vi "Dashboard Main.vi"() -> ()   [LabVIEW 2017]
uses:
  <vilib>/Utility/miscctls.llb/LVRowAndColumnTypeDef.ctl
  <vilib>/event_ctls.llb/eventvkey.ctl
  <vilib>/Rock Robotics/Network Tables/NT Read Numeric Array.vi
  <vilib>/Rock Robotics/Network Tables/NT Read Boolean Array.vi
  <vilib>/Rock Robotics/WPI/Dashboard/WPI_DashboardLogging Global.vi
panel:
  in  "Camera Settings Right":T1={"Frame Rate"=30, "Compression"=30, "Size"=1, "DB Camera Config"=FALSE} {"Frame Rate" scale=1.0..30.0; "Compression" scale=100.0..-1.0; "Size" items=["640x480", "320x240", "160x120"]}
  in  "Camera Name Right":string(combo)="No Camera Selection"
  out "Camera Info":cluster{"Mbps LED":bool, "Mbps":dbl, "fps":dbl} {"fps" format="%#.1g"; "Mbps" format="%#.1g"}
  in  "Camera Settings":T1={"Frame Rate"=30, "Compression"=30, "Size"=1, "DB Camera Config"=FALSE} {"Frame Rate" scale=1.0..30.0; "Compression" scale=100.0..-1.0; "Size" items=["640x480", "320x240", "160x120"]}
  in  "TCP":refnum<k5>
  in  "Rec Mode":enum32{"Stop", "Record", "Playback"}(radio)
  out "Robot IP":string
  out "Image Message":string="Timeout in Camera Communications"
  in  "Dashboard Tab":T2(tab)
  out "NT Connection":bool
  out "MotorChart R":cluster{"Numeric":dbl, "Numeric":dbl}(graph)
  out "MotorChart L":cluster{"Numeric":dbl, "Numeric":dbl}(graph)
  out "MotorSliders R":cluster{"MotorSlide1":dbl, "MotorSlide2":dbl} {"MotorSlide2" scale=-1.0..1.0 scale format="%#_2e"; "MotorSlide1" scale=-1.0..1.0 scale format="%#_2e"}
  out "MotorSliders L":cluster{"MotorSlide1":dbl, "MotorSlide2":dbl} {"MotorSlide2" scale=-1.0..1.0 scale format="%#_2e"; "MotorSlide1" scale=-1.0..1.0 scale format="%#_2e"}
  out "JS1 Z":dbl(slide) scale=-1.0..1.0 scale format="%#_2e"
  out "JS1 Graph":cluster{"X":dbl, "Y":dbl}[](graph)
  out "JS1 Buttons":T3
  out "JS2 Z":dbl(slide) scale=-1.0..1.0 scale format="%#_2e"
  out "JS2 Graph":cluster{"X":dbl, "Y":dbl}[](graph)
  out "JS2 Buttons":T3
  out "Mode":T4(ring)=enum."Auto Disabled"
  out "Gear State":string="Waiting...."
  out "Ramps":bool[](array[boolean])
  out "Camera Image Right":T5(plugin-control)
  in  "DB/String 9":string
  in  "DB/String 8":string
  in  "DB/String 7":string
  in  "DB/String 6":string
  in  "DB/String 5":string
  in  "DB/String 4":string
  in  "DB/String 3":string
  in  "DB/String 2":string
  in  "DB/String 1":string
  in  "DB/String 0":string
  in  "DB/Slider 0":dbl(slide) scale=0.0..5.0
  in  "DB/Slider 1":dbl(slide) scale=0.0..5.0
  in  "DB/Slider 2":dbl(slide) scale=0.0..5.0
  in  "DB/Slider 3":dbl(slide) scale=0.0..5.0
  out "DB/LED 3":bool
  out "DB/LED 2":bool
  out "DB/LED 1":bool
  out "DB/LED 0":bool
  in  "DB/Button 3":bool
  in  "DB/Button 2":bool
  in  "DB/Button 1":bool
  in  "DB/Button 0":bool caption="New Name"
  in  "Test Slider":dbl(slide) scale=0.0..100.0 scale format="%#_3g"
  in  "On/Off":bool caption="Solenoid"
  in  "Test Name":u16(ring) items=["Select the test to run..."]
  in  "Test Tree":string(tree)
  in  "Motor":cluster{"Value":dbl, "Enable":bool} {"Value" scale=-1.0..1.0 scale format="%#_3g"}
  out "Progress":T6 {"Test Progress" scale=0.0..100.0}
  in  "Rev/Fwd":cluster{"Forward":bool, "Reverse":bool}
  in  "Test Ring":u16(ring) items=["Monochrome", "Color"]
  out "Cmd Status":string
  in  "Execute Command":bool
  in  "Command Params":string[][](table)
  in  "Command Selection":i32(listbox)
  in  "CheckList":i32(listbox)
  out "Tree":string(tree)
  out "new picture":picture
  in  "Starting Pos":i16(slide)=128 scale=340.0..50.0
  in  "Right String":string
  in  "Left String":string
  in  "Load Left Auto":bool
  in  "Save Left Auto":bool
  in  "Save Right Auto":bool
  in  "Load Right Auto":bool
  in  "Select Auto":string(combo)="Select Autonomous ..."
  out "Camera Image":T5(plugin-control)
  out "Background":bool
  in  "Camera Name":string(combo)="No Camera Selection"
  # "HW"
  # "HW"
  # "Joysticks"
  # "Drive Motors"
  # "Front"
  # "Right"
  # "Left"
  # "Back"
  # "This tab is a great place for autonomous settings and robot-specific values.\nPlace controls and indicators inside this tab and match name to\nDashboard Variables on robot. You can also delete this comment."
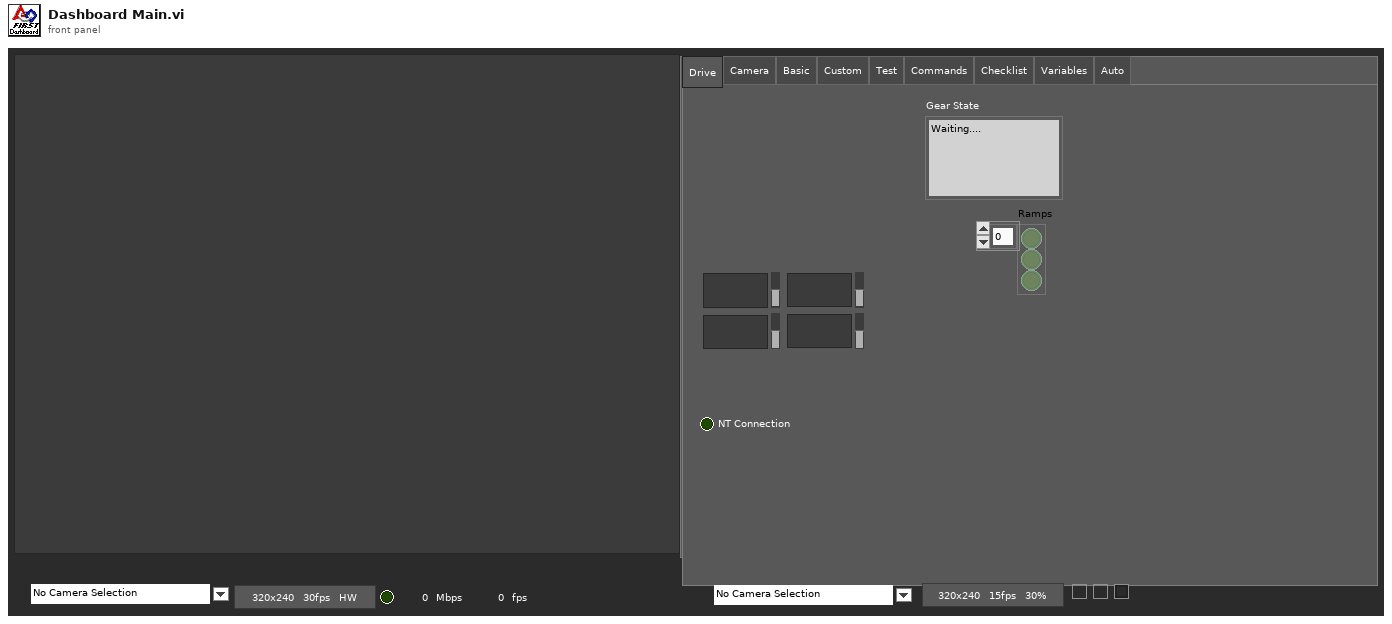
[diagram p1: front panel]
types:
  T1 = cluster{"Frame Rate":i32, "Compression":i32, "Size":u16, "DB Camera Config":bool}
  T2 = enum32{"Drive", "Camera", "Basic", "Custom", "Test", "Commands", "Checklist", "Variables", "Auto"}
  T3 = cluster{bool, bool, bool, bool, bool, bool, bool, bool, bool, bool, bool, bool}
  T4 = enum8{"Tele-Op Disabled", "Tele-Op Enabled", "Auto Disabled", "Auto Enabled", "Test Disabled", "Test Enabled", "Disconnected", "No Code", "E-Stop"}
  T5 = typedef "IMAQ Image.ctl" = refnum<image>
  T6 = cluster{"Test Progress":u8, "Test Progress Text":string}
  T7 = cluster{"Save Path":path, "Interval (s)":dbl, "Keep":i32}
  T8 = enum32{"Drive", "Camera", "Basic", "Custom", "Test", "Commands", "Checklist", "Variables"}
  T9 = typedef "Image Type" = u32
  T10 = cluster{"IDs":cluster{"RPC field ID":u16, "Unique ID":u16}, "String":string}
  T11 = cluster{"Error Strings":string, "Disable Counts":cluster{u16, u16}, "Rail Faults":cluster{u16, u16, u16}, "Robot IP":string, "DB Mode":u8, "Event Info":cluster{"Name":string, "Type":u8, "Number":u16, "Replay":u8}}
  T12 = cluster{"Storage":cluster{"Disk Free":u64, "RAM Block":u32, "RAM free":u32}, "CPU Utilization":cluster{"CPU % ISR":sgl, "CPU % Time Crit":sgl, "CPU % Timed Str":sgl, "CPU % High":sgl, "CPU % Above":sgl, "CPU % Normal":sgl, "CPU % Low":sgl}, "CAN":cluster{"% Bus Utilization":sgl, "Bus Off Cnt":u32, "TX_FIFO Full Cnt":u32, "Receive Error Cnt":u8, "Transmit Error Cnt":u8}, "HID":cluster{"HID Outputs":u32, "Rumble Low":u16, "Rumble High":u16}[]}
  T13 = cluster{"Status bits":cluster{"Test Mode":bool, "Autonomous":bool, "Enabled":bool, "Code Start":bool, "Brownout":bool, "Reserved 2":bool, "Reserved 3":bool, "E-Stop":bool}, "Code Trace":cluster{"Disabled":bool, "TeleOp":bool, "Auto":bool, "Test":bool}, "Controller Type":enum16{"unknown", "cRIO", "roboRio"}, "Code?":enum16{"unknown", "noCode", "code"}, "Battery V":dbl}
  T14 = cluster{"Control Bits":cluster{"TestMode":bool, "Autonomous":bool, "Enabled":bool, "FMS Present":bool, bool, bool, bool, "E-Stop":bool}, "Team Station ":u8, "Countdown":sgl, "Joystick Values":cluster{"Axes":dbl[], "Buttons":bool[], "POVs":i16[]}[]}
  T15 = cluster{"Axes":dbl[], "Buttons":bool[], "POVs":i16[]}[]
  T16 = cluster{"Axes":dbl[], "Buttons":bool[], "POVs":i16[]}
  T17 = cluster{"Buttons[0]":bool, "Buttons[1]":bool, "Buttons[2]":bool, "Buttons[3]":bool, "Buttons[4]":bool, "Buttons[5]":bool, "Buttons[6]":bool, "Buttons[7]":bool, "Buttons[8]":bool, "Buttons[9]":bool, "Buttons[10]":bool, "Buttons[11]":bool}
  T18 = typedef "LVBoundsTypeDef.ctl" = cluster{"Width":u32, "Height":u32}
  T19 = cluster{"Camera Image":refnum<vi>, "Dashboard Tab":refnum<vi>, "Background":refnum<vi>, "Rec Mode":refnum<vi>, "Test Slider":refnum<vi>, "On/Off ":refnum<vi>, "Test Ring":refnum<vi>, "Rev/Fwd":refnum<vi>, "Test Name":refnum<vi>, "Motor":refnum<vi>, "Progress":refnum<vi>, "CheckList":refnum<vi>, "Tree":refnum<vi>, "Test Tree":refnum<vi>, "Command Params":refnum<vi>, "Command Selection":refnum<vi>, "Execute Command":refnum<vi>, "Cmd Status":refnum<vi>, "Camera Settings":refnum<vi>, "Camera Name":refnum<vi>, "Camera Info":refnum<vi>, "Camera Settings Right":refnum<vi>, "Camera Name Right":refnum<vi>, "Camera Image Right":refnum<vi>}
  T20 = cluster{"Camera Name":string, string, "Saved DB Images Info":cluster{"Save Path":path, "Interval (s)":dbl, "Keep":i32}}
  T21 = cluster{"Camera Name Right":string, string, "Saved DB Images Info":cluster{"Save Path":path, "Interval (s)":dbl, "Keep":i32}}
  T22 = cluster{"Operation":enum16{"Update", "Clear"}, "Color Box":u32}[]
  T23 = typedef "eventvkey.ctl" = enum16{"ASCII", "Enter", "Return", "Shift", "Ctrl", "Alt", "Cmd", "Opt", "Caps", "NumLock", "Clear", "Break", "Up", "Down", "Left", "Right", "Insert", "Delete", "Home", "End", "PageUp", "PageDown", "Escape", "Help", "Pause", "ScrollLock", "F1", "F2", "F3", "F4", "F5", "F6", "F7", "F8", "F9", "F10", "F11", "F12", "F13", "F14", "F15", "F16", "F17", "F18", "F19", "F20", "F21", "F22", "F23", "F24", "Play", "VolumeUp", "VolumeDown", "Mute", "Two Byte Char"}
  T24 = cluster{"Image Size":bool, "Image Type":bool, "Pixel Value":bool, "ROI Information":bool, "Zoom Factor":bool}
  T25 = cluster{"Operation":enum16{"Update", "Clear"}, "Color Box":u32}
  T26 = typedef "LVRowAndColumnTypeDef.ctl" = cluster{"Row":i32, "Column":i32}
  T27 = cluster{"Shift":bool, "Ctrl":bool, "Alt":bool, "Cmd":bool, "Opt":bool}
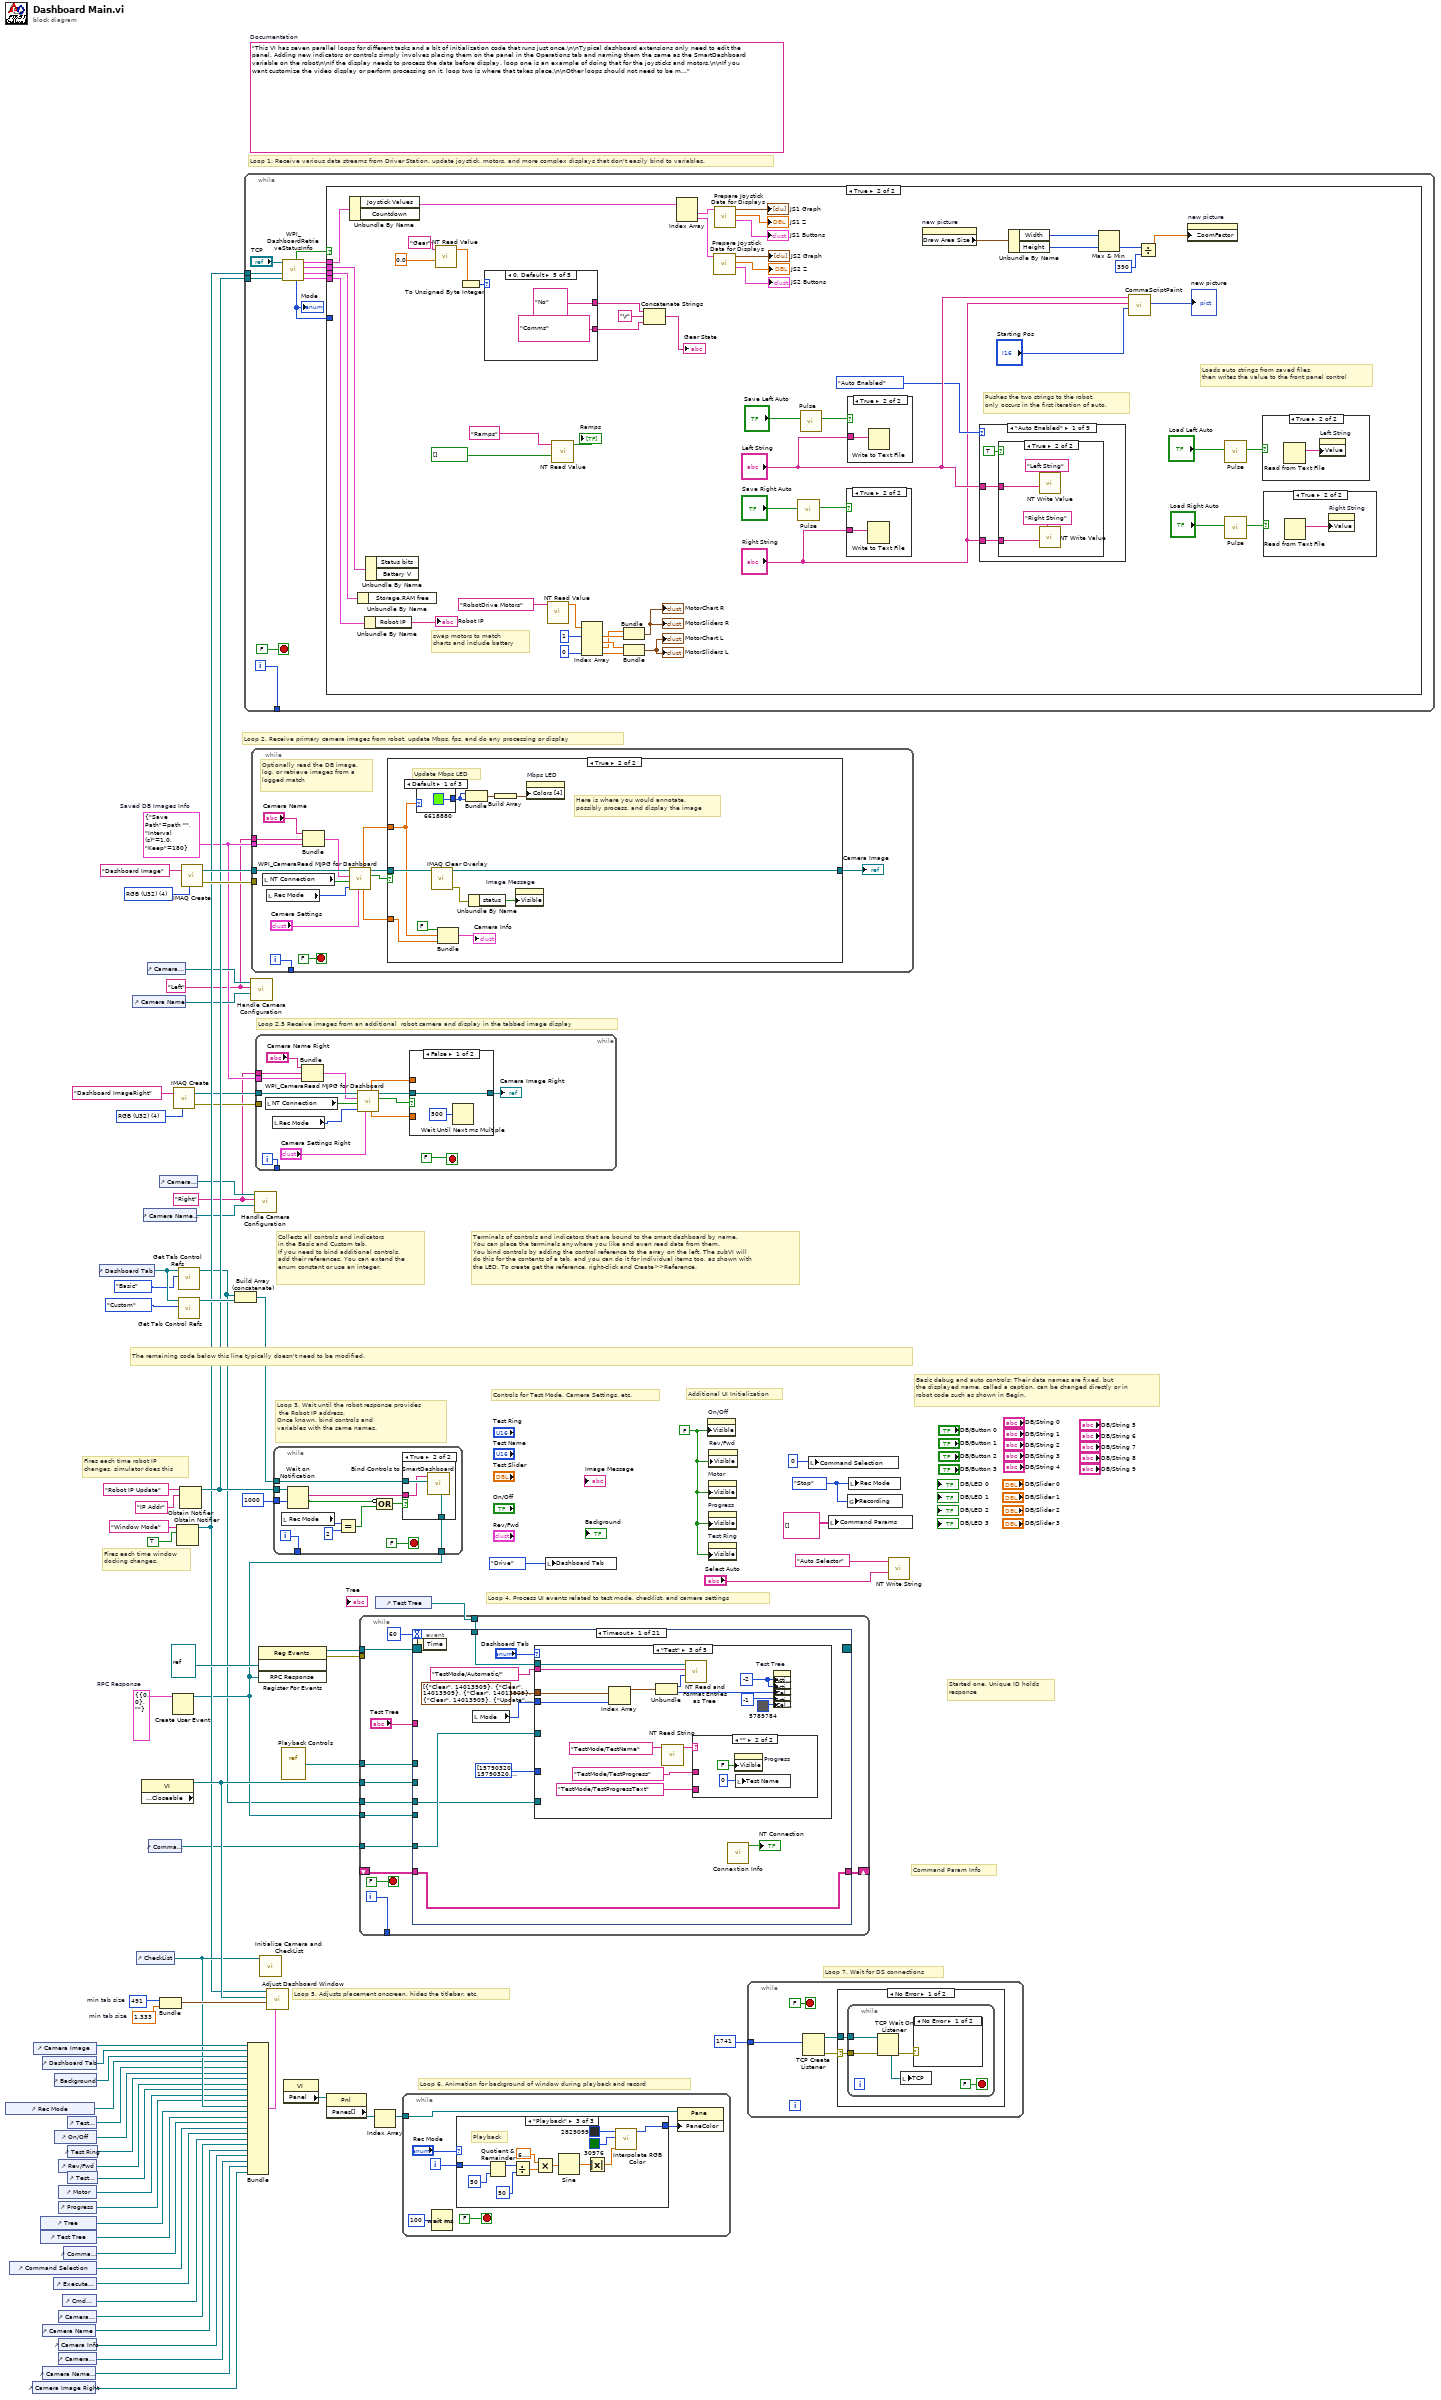
[diagram p0: block diagram]
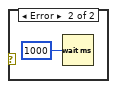
[diagram p3: hidden frame]
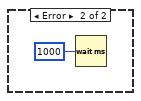
[diagram p4: hidden frame]
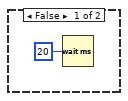
[diagram p5: hidden frame]
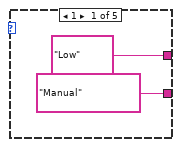
[diagram p19: hidden frame]
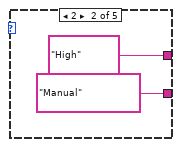
[diagram p20: hidden frame]
diagram:
  w3 = T7 {"Save Path"=path "", "Interval (s)"=1.0, "Keep"=180}  # Saved DB Images Info
  w2 = "Right"
  w1 = "Left"
  w13 = T9 4 items=["Grayscale (U8)", "Grayscale (I16)", "Grayscale (SGL)", "Complex (CSG)", "RGB (U32)", "HSL (U32)", "RGB (U64)"] ("Image Type")
  w29 = T10 {"IDs"={"RPC field ID"=0, "Unique ID"=0}, "String"=""}  # RPC Response
  w52 = 491  # min tab size
  w51 = 1.333  # min tab size
  w59 = enum32{"Stop", "Record", "Playback"}."Stop" ("Rec Mode")
  w36 = FALSE ("Visible")
  (unwired) "This VI has seven parallel loops for different tasks and a bit of initialization code that runs just once.\n\nTypical dashboard extensions only need to edit the panel. Adding new indicators or controls simply involves placing them on the panel in the Operations tab and naming them the same as the SmartDashboard variable on the robot\n\nIf the display needs to process the data before display, loop one is an example of doing that for the joysticks and motors.\n\nIf you want customize the video display or perform processing on it, loop two is where that takes place.\n\nOther loops should not need to be modified. They are pretty standard, and document the task they perform."  # Documentation
  w76 = T9 4 items=["Grayscale (U8)", "Grayscale (I16)", "Grayscale (SGL)", "Complex (CSG)", "RGB (U32)", "HSL (U32)", "RGB (U64)"] ("Image Type")
  # "Loop 2.5 Receive images from an additional  robot camera and display in the tabbed image display"
  # "Command Param Info"
  # "Started one, Unique ID holds\nresponse"
  # "Loop 7. Wait for DS connections"
  # "Basic debug and auto controls: Their data names are fixed, but\nthe displayed name, called a caption, can be changed directly or in\nrobot code such as shown in Begin."
  # "Controls for Test Mode, Camera Settings, etc."
  # "Additional UI Initialization"
  # "Loop 6. Animation for background of window during playback and record"
  # "Fires each time robot IP\nchanges, simulator does this"
  # "Fires each time window\ndocking changes."
  # "Collects all controls and indicators\nin the Basic and Custom tab.\nIf you need to bind additional controls,\nadd their references. You can extend the\nenum constant or use an integer."
  # "The remaining code below this line typically doesn't need to be modified."
  # "Loop 4. Process UI events related to test mode, checklist, and camera settings"
  # "Terminals of controls and indicators that are bound to the smart dashboard by name.\nYou can place the terminals anywhere you like and even read data from them.\nYou bind controls by adding the control reference to the array on the left. The subVI will\ndo this for the contents of a tab, and you can do it for individual items too, as shown with\nthe LED. To create get the reference, right-click and Create>>Reference."
  # "Loop 3. Wait until the robot response provides\n the Robot IP address.\nOnce known, bind controls and\nvariables with the same names."
  # "Loop 5. Adjusts placement onscreen, hides the titlebar, etc."
  # "Loop 1. Receive various data streams from Driver Station, update joystick, motors, and more complex displays that don't easily bind to variables."
  # "Loop 2. Receive primary camera images from robot, update Mbps, fps, and do any processing or display"
  n1 = control-ref of="Rec Mode"() -> (w42:refnum<vi>)
  n2 = control-ref of="Command Selection"() -> (w28:refnum<vi>)
  n3 = control-ref of="Camera Image Right"() -> (w6:refnum<vi>)
  n4 = control-ref of="Camera Image"() -> (w54:refnum<vi>)
  n5 = control-ref of="Tree"() -> (w46:refnum<vi>)
  n6 = control-ref of="Test Tree"() -> (w45:refnum<vi>)
  n7 = control-ref of="Dashboard Tab"() -> (w53:refnum<vi>)
  n8 = control-ref of="Camera Name"() -> (w19:refnum<vi>)
  n9 = control-ref of="Camera Name Right"() -> (w7:refnum<vi>)
  n10 = control-ref of="Execute Command"() -> (w30:refnum<vi>)
  n11 = control-ref of="Background"() -> (w49:refnum<vi>)
  n12 = control-ref of="On/Off"() -> (w40:refnum<vi>)
  n13 = control-ref of="Progress"() -> (w37:refnum<vi>)
  n14 = control-ref of="Camera Settings"() -> (w20:refnum<vi>)
  n15 = control-ref of="Camera Info"() -> (w18:refnum<vi>)
  n16 = control-ref of="Camera Settings Right"() -> (w8:refnum<vi>)
  n17 = control-ref of="Rev/Fwd"() -> (w38:refnum<vi>)
  n18 = control-ref of="Motor"() -> (w43:refnum<vi>)
  n19 = control-ref of="Cmd Status"() -> (w24:refnum<vi>)
  n20 = control-ref of="Command Params"() -> (w31:refnum<vi>)
  n21 = control-ref of="Test Slider"() -> (w41:refnum<vi>)
  n22 = control-ref of="Test Ring"() -> (w39:refnum<vi>)
  n23 = control-ref of="Test Name"() -> (w44:refnum<vi>)
  n24 = control-ref of="Dashboard Tab"() -> (w57:refnum<vi>)
  n25 = control-ref of="Camera Name"() -> (w21:refnum<vi>)
  n26 = control-ref of="CheckList"() -> (w47:refnum<vi>)
  n27 = property class="VI" props=["Front Panel.Closeable"]() -> (reference out=w58:refnum<vi>)  [unwired: 2 in, 2 out]
  n28 = control-ref of="Camera Name Right"() -> (w9:refnum<vi>)
  n29 = control-ref of="Camera Settings"() -> (w22:refnum<vi>)
  n30 = control-ref of="Command Params"() -> (w23:refnum<vi>)
  n31 = control-ref of="Camera Settings Right"() -> (w10:refnum<vi>)
  n32 = Bundle("min tab size"=w52, "min tab size"=w51) -> (w50:cluster{"min tab size":i32, "min tab size":dbl})  [unwired: 1 in]
  n33 = Create User Event(user event datatype=w29) -> (user event=w25:refnum<user-event>)  [unwired: 1 in, 1 out]
  n34 = call "IMAQ Create"("Image Name"="Dashboard ImageRight", "Image Type"=w13) -> ("New Image"=w12:T5, "error out"=w11:errorcluster)  [unwired: 2 in, 1 out]
  n35 = Obtain Notifier(name (unnamed)="Window Mode", notification data type=TRUE) -> (notifier out=w34:refnum<notifier>)  [unwired: 2 in, 2 out]
  n36 = call <vilib>:"Get Tab Control Refs.vi"("Page Index"=T8."Basic" ("Dashboard Tab"), "TabControl in"=w57) -> ("ControlsOnPage"=w17:refnum<vi>[])  [unwired: 9 in]
  n37 = call <vilib>:"Get Tab Control Refs.vi"("Page Index"=T8."Custom" ("Dashboard Tab"), "TabControl in"=w57) -> ("ControlsOnPage"=w56:refnum<vi>[])  [unwired: 9 in]
  n38 = Obtain Notifier(name (unnamed)="Robot IP Update", notification data type="IP Addr" ("name (unnamed)")) -> (notifier out=w35:refnum<notifier>)  [unwired: 2 in, 2 out]
  n39 = call "IMAQ Create"("Image Name"="Dashboard Image", "Image Type"=w76) -> ("New Image"=w74:T5, "error out"=w73:errorcluster)  [unwired: 2 in, 1 out]
  n40 = Build Array (concatenate)(w17, w56) -> (w55:refnum<vi>[])
  n41 = while {
    tunnel: [w86] -> _
    tunnel: w35 -> [w80]
    tunnel: w34 -> [w77]
    i -> [w86]
    stop <- FALSE stop-if-true
    n42 = call <vilib>:"WPI_DashboardRetrieveStatusInfo.vi"("Binding Refnum"=w80, "Window Mode Notifier"=w77, "TCP Cnx"="TCP") -> ("Power and Errors"=w81:T11, "Robot Metrics"=w84:T12, "Status Info"=w85:T13, "Control Info"=w82:T14, "Robot Mode"=w79:T4, "Process?"=w83:bool)  [unwired: 3 in]
    "Mode" <- w79
    n43 = case shown="True" w83 {
      tunnel: w85 -> [_ w142]
      tunnel: w84 -> [_ w141]
      tunnel: w82 -> [_ w140]
      tunnel: w81 -> [_ w139]
      tunnel: w79 -> [_ _]
      frame False {
        n44 = Wait (ms)(milliseconds to wait=u32 20) -> ()  [unwired: 1 out]
      }
      frame True {
        # "Pushes the two strings to the robot,\nonly occurs in the first iteration of auto."
        # "Loads auto strings from saved files,\nthen writes the value to the front panel control"
        # "swap motors to match\ncharts and include battery"
        n45 = Unbundle By Name(w140) -> ("Joystick Values"=w130:T15)  [unwired: 1 out]
        n46 = Unbundle By Name(w141) -> ()  [unwired: 1 out]
        n47 = Unbundle By Name(w139) -> ("Robot IP"=→"Robot IP":string)
        n48 = Unbundle By Name(w142) -> ()  [unwired: 2 out]
        n49 = call-poly <vilib>:"NT Read Value.vi"("Default Value"=0.0, "Name"="Gear") -> ("Numeric"=w117:dbl)  [unwired: 8 in, 1 out]
        n50 = To Unsigned Byte Integer(number=w117) -> (unsigned 8bit integer=w118:u8)
        n51 = case shown="0, Default" w118 {
          tunnel: ["Low" "High" "Low" "High" "No"] -> w114
          tunnel: ["Manual" "Manual" "Automatic" "Automatic" "Comms"] -> w112
          frame 1 {
          }
          frame 2 {
          }
          frame 3 {
          }
          frame 4 {
          }
          frame 0, Default {
          }
        }
        n52 = call-poly <vilib>:"NT Read Value.vi"("Name"="RobotDrive Motors") -> ("Numeric Array"=w120:dbl[])  [unwired: 9 in, 1 out]
        n53 = call-poly <vilib>:"NT Read Value.vi"("Default Value"=bool[] [], "Name"="Ramps") -> ("Boolean Array"=→"Ramps":bool[])  [unwired: 8 in, 1 out]
        n54 = Index Array(array=w120, index #1=1, index #4=0) -> (element #1=w134:dbl, element #2=w135:dbl, element #3=w133:dbl, element #4=w138:dbl)  [unwired: 2 in]
        n55 = Bundle("Numeric"=w133, "Numeric"=w134) -> (→"MotorChart R" →"MotorSliders R":cluster{"Numeric":dbl, "Numeric":dbl})  [unwired: 1 in]
        n56 = Bundle("Numeric"=w135, "Numeric"=w138) -> (→"MotorChart L" →"MotorSliders L":cluster{"Numeric":dbl, "Numeric":dbl})  [unwired: 1 in]
        n57 = Concatenate Strings(w114, "\r", w112) -> (→"Gear State":string)
        n58 = Index Array(array=w130) -> (element #1=w129:T16, element #2=w125:T16)  [unwired: 2 in]
        n59 = call "Prepare Joystick Data for Displays.vi"("Joystick Values"=w125) -> ("Buttons"=→"JS2 Buttons":T17, "Z Axis"=→"JS2 Z":dbl, "Cartesian Data"=→"JS2 Graph":cluster{"X axis":dbl, "X axis":dbl}[])  [unwired: 8 in]
        n60 = call "Prepare Joystick Data for Displays.vi"("Joystick Values"=w129) -> ("Buttons"=→"JS1 Buttons":T17, "Z Axis"=→"JS1 Z":dbl, "Cartesian Data"=→"JS1 Graph":cluster{"X axis":dbl, "X axis":dbl}[])  [unwired: 8 in]
        n61 = call "Pulse.vi"("Input"="Save Right Auto") -> ("Output"=w105:bool)  [unwired: 10 in]
        n62 = call "Pulse.vi"("Input"="Save Left Auto") -> ("Output"=w101:bool)  [unwired: 10 in]
        n63 = case shown="True" w105 {
          tunnel: "Right String" -> [_ w150]
          frame False {
          }
          frame True {
            n64 = Write to Text File(text=w150) -> ()  [unwired: 3 in, 3 out]
          }
        }
        n65 = case shown="True" w101 {
          tunnel: "Left String" -> [_ w153]
          frame False {
          }
          frame True {
            n66 = Write to Text File(text=w153) -> ()  [unwired: 3 in, 3 out]
          }
        }
        n67 = property on="new picture" class="Pict"() -> ("Draw Area Size"=w93:T18)  [unwired: 2 in, 2 out]
        n68 = case shown="\"Auto Enabled\"" T4."Auto Enabled" ("Robot Mode") {
          tunnel: "Left String" -> [w145 _ _ _ _ _ _ _ _]
          tunnel: "Right String" -> [w144 _ _ _ _ _ _ _ _]
          frame "Auto Enabled" {
            n69 = case shown="True" TRUE {
              tunnel: w145 -> [_ w149]
              tunnel: w144 -> [_ w148]
              frame False {
              }
              frame True {
                n70 = call-poly <vilib>:"NT Write Value.vi"("String"=w149, "Name"="Left String") -> ()  [unwired: 9 in, 1 out]
                n71 = call-poly <vilib>:"NT Write Value.vi"("String"=w148, "Name"="Right String") -> ()  [unwired: 9 in, 1 out]
              }
            }
          }
          frame "Test Disabled" {
          }
          frame "Test Enabled" {
          }
          frame "Disconnected" {
          }
          frame "No Code" {
          }
          frame "E-Stop" {
          }
          frame "Auto Disabled" {
          }
          frame "Tele-Op Enabled" {
          }
          frame "Tele-Op Disabled" {
          }
        }
        n72 = Unbundle By Name(w93) -> ("Width"=w97:u32, "Height"=w96:u32)
        n73 = Max & Min(x=w97, y=w96) -> (min(x,y)=w95:u32)  [unwired: 1 out]
        n74 = call "CommaScriptPaint.vi"("Starting Pos"="Starting Pos", "string 2"="Right String", "string"="Left String") -> ("new picture"=→"new picture":picture)  [unwired: 7 in, 1 out]
        n75 = Divide(x=w95, y=u32 390) -> (x/y=w92:dbl)
        n76 = property on="new picture" class="Pict"("ZoomFactor"=w92) -> ()  [unwired: 2 in, 2 out]
        n77 = call "Pulse.vi"("Input"="Load Left Auto") -> ("Output"=w102:bool)  [unwired: 10 in]
        n78 = call "Pulse.vi"("Input"="Load Right Auto") -> ("Output"=w108:bool)  [unwired: 10 in]
        n79 = case shown="True" w102 {
          frame False {
          }
          frame True {
            n80 = Read from Text File() -> (text=w152:string)  [unwired: 4 in, 3 out]
            n81 = property on="Left String" class="Str"("Value"=w152) -> ()  [unwired: 2 in, 2 out]
          }
        }
        n82 = case shown="True" w108 {
          frame False {
          }
          frame True {
            n83 = Read from Text File() -> (text=w151:string)  [unwired: 4 in, 3 out]
            n84 = property on="Right String" class="Str"("Value"=w151) -> ()  [unwired: 2 in, 2 out]
          }
        }
      }
    }
  }
  n85 = Bundle("Camera Image"=w54, "Dashboard Tab"=w53, "Background"=w49, "Rec Mode"=w42, "Test Slider"=w41, "On/Off"=w40, "Test Ring"=w39, "Rev/Fwd"=w38, "Test Name"=w44, "Motor"=w43, "Progress"=w37, "CheckList"=w47, "Tree"=w46, "Test Tree"=w45, "Command Params"=w31, "Command Selection"=w28, "Execute Command"=w30, "Cmd Status"=w24, "Camera Settings"=w20, "Camera Name"=w19, "Camera Info"=w18, "Camera Settings Right"=w8, "Camera Name Right"=w7, "Camera Image Right"=w6) -> (w48:T19)  [unwired: 1 in]
  n86 = call "Handle Camera Configuration.vi"("CameraNameRef"=w21, "Display Name"=w1, "ClusterRef"=w22) -> ()  [unwired: 9 in]
  n87 = while {
    tunnel: w74 -> [w176]
    tunnel: w73 -> [_]
    tunnel: [w177] -> _
    tunnel: w3 -> [w167]
    tunnel: w1 -> [w164]
    i -> [w177]
    stop <- FALSE stop-if-true
    # "Optionally read the DB image,\nlog, or retrieve images from a\nlogged match"
    n88 = local read "NT Connection"() -> (w168:bool)
    n89 = local read "Rec Mode"() -> (w172:enum32{"Stop", "Record", "Playback"})
    n90 = Bundle("Camera Name"="Camera Name", w164, "Saved DB Images Info"=w167) -> (w166:T20)  [unwired: 1 in]
    n91 = call <vilib>:"WPI_CameraRead MJPG for Dashboard.vi"("Camera Settings"="Camera Settings", "Rec Mode"=w172, "NT Connection"=w168, "Capture Info"=w166, "Refnum in"=w176) -> ("Active"=w174:bool, "Refnum out"=w175:T5, "FPS"=w173:dbl, "Bandwidth (Mbps)"=w171:dbl)  [unwired: 3 in]
    n92 = case shown="True" w174 {
      tunnel: w175 -> [w179 w190]
      tunnel: w171 -> [_ w187]
      tunnel: w173 -> [_ w188]
      tunnel: [w179 w184] -> w169
      frame False {
        w181 = u32 1985280 ("Color Box")
        # "Sleep for 500ms"
        n93 = Bundle("Color Box"=w181, "Color Box"=w181) -> (w182:cluster{"Color Box":u32, "Color Box":u32})  [unwired: 1 out]
        n94 = Build Array(w182) -> (w180:cluster{"Color Box":u32, "Color Box":u32}[])
        n95 = property on="Mbps LED" class="Bool (strict)"("Colors [4]"=w180) -> ()  [unwired: 2 in, 2 out]
        n96 = Wait Until Next ms Multiple(millisecond multiple=u32 500) -> ()  [unwired: 1 out]
      }
      frame True {
        # "Here is where you would annotate,\npossibly process, and display the image"
        # "Update Mbps LED"
        n97 = case shown="Default" w187 {
          tunnel: [u32 6618880 ("Color Box") u32 16776722 ("Color Box") u32 16716800 ("Color Box")] -> w191
          frame Default {
          }
          frame 4, 5 {
          }
          frame 6.. {
          }
        }
        n98 = call "IMAQ Clear Overlay"("Image"=w190) -> ("error out"=w193:errorcluster, "Image Out"=w184:T5)  [unwired: 2 in, 7 out]
        n99 = Bundle(FALSE, "Bandwidth (Mbps)"=w187, "FPS"=w188) -> (→"Camera Info":cluster{bool, "Bandwidth (Mbps)":dbl, "FPS":dbl})  [unwired: 1 in]
        n100 = Bundle("Color Box"=w191, "Color Box"=w191) -> (w192:cluster{"Color Box":u32, "Color Box":u32})  [unwired: 1 out]
        n101 = Unbundle By Name(w193) -> ("status"=w194:bool)
        n102 = Build Array(w192) -> (w189:cluster{"Color Box":u32, "Color Box":u32}[])
        n103 = property on="Image Message" class="Str"("Visible"=w194) -> ()  [unwired: 2 in, 2 out]
        n104 = property on="Mbps LED" class="Bool (strict)"("Colors [4]"=w189) -> ()  [unwired: 2 in, 2 out]
      }
    }
    "Camera Image" <- w169
  }
  n105 = call "Handle Camera Configuration.vi"("CameraNameRef"=w9, "Display Name"=w2, "ClusterRef"=w10) -> ()  [unwired: 9 in]
  n106 = while {
    tunnel: w12 -> [w212]
    tunnel: w11 -> [_]
    tunnel: [w207] -> _
    tunnel: w3 -> [w201]
    tunnel: w2 -> [w198]
    i -> [w207]
    stop <- FALSE stop-if-true
    n107 = local read "NT Connection"() -> (w202:bool)
    n108 = local read "Rec Mode"() -> (w211:enum32{"Stop", "Record", "Playback"})
    n109 = Bundle("Camera Name Right"="Camera Name Right", w198, "Saved DB Images Info"=w201) -> (w200:T21)  [unwired: 1 in]
    n110 = call <vilib>:"WPI_CameraRead MJPG for Dashboard.vi"("Camera Settings"="Camera Settings Right", "Rec Mode"=w211, "NT Connection"=w202, "Capture Info"=w200, "Refnum in"=w212) -> ("Active"=w206:bool, "Refnum out"=w209:T5, "FPS"=w204:dbl, "Bandwidth (Mbps)"=w205:dbl)  [unwired: 3 in]
    n111 = case shown="False" w206 {
      tunnel: w209 -> [w213 w215]
      tunnel: w205 -> [_ _]
      tunnel: w204 -> [_ _]
      tunnel: [w213 w215] -> w203
      frame False {
        n112 = Wait Until Next ms Multiple(millisecond multiple=u32 500) -> ()  [unwired: 1 out]
      }
      frame True {
      }
    }
    "Camera Image Right" <- w203
  }
  n113 = register-events(refnum<vi> refnum, w25) -> (reference out=w63:refnum<event-registration>, error out=w62:errorcluster)  [unwired: 2 in]
  n114 = call "Initialize Camera and CheckList.vi"("ListBox in"=w47) -> ()  [unwired: 11 in]
  n115 = call "Adjust Dashboard Window.vi"("Sizing Refnums"=w48, "Size Constraints"=w50, "VI"=w58, "WIn Mode"=w34) -> ()  [unwired: 8 in]
  n116 = while {
    tunnel: w55 -> [w227]
    tunnel: w35 -> [w225]
    tunnel: [w223] -> _
    tunnel: u32 1000 ("milliseconds to wait") -> [w222]
    tunnel: w25 -> [w216]
    i -> [w223]
    stop <- FALSE stop-if-true
    n117 = local read "Rec Mode"() -> (w218:enum32{"Stop", "Record", "Playback"})
    n118 = Wait on Notification(notifier=w225, timeout in ms (-1)=w222) -> (notification=w224:string, timed out?=w220:bool)  [unwired: 2 in, 2 out]
    n119 = Equal?(x=w218, y=u16 2 ("Rec Mode")) -> (x = y?=w219:bool)
    n120 = Compound Arithmetic op=OR(invert w220, w219) -> (w221:bool)
    n121 = case shown="True" w221 {
      tunnel: w227 -> [_ w230]
      tunnel: w224 -> [_ w229]
      tunnel: w216 -> [_ w228]
      frame False {
      }
      frame True {
        n122 = call <vilib>:"Bind Controls to SmartDashboard.vi"("RPC ref"=w228, "Bound Control Refs"=w230, "Server IP Address"=w229) -> ()  [unwired: 9 in]
      }
    }
  }
  n123 = vi-ref "Playback Controls.vi"() -> (w64:refnum<vi>)
  n124 = property class="VI"() -> ("Panel"=w66:refnum<vi>)  [unwired: 2 in, 2 out]
  n125 = property class="Pnl"(reference=w66) -> ("Panes[]"=w67:refnum<vi>[])  [unwired: 1 in, 2 out]
  n126 = Index Array(array=w67) -> (element=w65:refnum<vi>)  [unwired: 1 in]
  n127 = control-ref of="Test Tree"() -> (w68:refnum<vi>)
  n128 = while {
    tunnel: [w240] -> _
    tunnel: w68 -> [w239]
    tunnel: w64 -> [w238]
    tunnel: w63 -> [w237]
    tunnel: w62 -> [_]
    tunnel: w58 -> [w236]
    tunnel: w25 -> [w235]
    tunnel: w23 -> [w234]
    shift-right: [w233] -> _
    shift-left: _ -> [w232]
    tunnel: w17 -> [w231]
    i -> [w240]
    stop <- FALSE stop-if-true
    n129 = event shown="[0] Timeout" {
      selector: w237 -> [_ _ _ _ _ _ _ _ _ _ _ _ _ _ _ _ _ _ _ _ _]
      dyn-events: [_ _ _ _ _ _ _ _ _ _ _ _ _ _ _ _ w500 _ _ _ _] -> _
      timeout: u32 60 ("milliseconds to wait") -> [_ _ _ _ _ _ _ _ _ _ _ _ _ _ _ _ _ _ _ _ _]
      tunnel: w239 -> [w252 _ _ _ _ _ _ _ _ _ _ _ _ _ _ _ _ _ _ _ _]
      tunnel: "Test Tree" -> [_ _ _ _ _ _ _ _ _ _ _ w467 w475 w477 w481 w489 _ _ _ _ _]
      tunnel: w238 -> [_ _ _ _ _ _ _ _ _ _ _ _ _ _ _ _ w502 _ w520 _ _]
      tunnel: w236 -> [_ _ _ _ _ _ _ _ _ _ _ _ _ _ _ _ w498 _ _ _ _]
      tunnel: w235 -> [_ _ _ _ _ _ _ _ _ _ _ _ _ _ _ _ w496 _ _ _ _]
      tunnel: w234 -> [w247 _ _ _ _ _ w418 _ _ _ _ _ _ _ _ _ _ _ _ _ _]
      tunnel: [w246 w295 w397 w402 w411 w415 w416 w425 w435 w442 w454 w466 w473 w476 w480 w488 w495 w515 w517 w521 w534] -> w233
      tunnel: w232 -> [w246 w295 w397 w402 w411 w415 w416 _ _ w442 w454 w466 w473 w476 w480 w488 w495 w515 w517 w521 w534]
      tunnel: w231 -> [w244 _ _ _ _ _ _ _ _ _ _ _ _ _ _ _ _ _ _ _ _]
      event Timeout {
        n130 = event-data() -> ()  [unwired: 1 in, 1 out]
        n131 = local read "Mode"() -> (w249:T4)
        n132 = case shown="\"Test\"" "Dashboard Tab" {
          tunnel: w252 -> [_ _ w268 _ _]
          tunnel: "TestMode/Automatic/" ("Name Pattern") -> [_ _ w267 _ _]
          tunnel: T22 [{"Operation"=enum."Clear", "Color Box"=14013909}, {"Operation"=enum."Clear", "Color Box"=14013909}, {"Operation"=enum."Clear", "Color Box"=14013909}, {"Operation"=enum."Clear", "Color Box"=14013909}, {"Operation"=enum."Update", "Color Box"=14013909}, {"Operation"=enum."Update", "Color Box"=16777215}, {"Operation"=enum."Clear", "Color Box"=14013909}, {"Operation"=enum."Clear", "Color Box"=14013909}, {"Operation"=enum."Clear", "Color Box"=14013909}] -> [_ _ w260 _ w288]
          tunnel: w249 -> [_ _ w259 _ w287]
          tunnel: u32[] [15790320, 15790320, 15790320, 15790320, 16777215, 16777215, 15790320, 15790320, 15790320] -> [_ _ _ _ w293]
          tunnel: w247 -> [_ _ _ _ w281]
          tunnel: w244 -> [_ w254 _ _ _]
          frame "Custom", Default {
          }
          frame "Basic" {
            n133 = call <vilib>:"WPI_DashboardUpdateNames.vi"("Controls on Tab"=w254) -> ()  [unwired: 11 in]
          }
          frame "Test" {
            w266 = -2 ("Active Item:Row Number")
            n134 = Index Array(array=w260, index=w259) -> (element=w261:T25)
            n135 = Unbundle(w261) -> ("Operation"=w262:enum16{"Update", "Clear"}, "Color Box"=w263:u32)
            n136 = call <vilib>:"NT Read String.vi"("Name"="TestMode/TestName") -> ("String"=w257:string)  [unwired: 9 in, 1 out]
            n137 = call <vilib>:"NT Read and Format Entries as Tree.vi"("Operation"=w262, "Name Pattern"=w267, "Tree Refnum"=w268) -> ()  [unwired: 7 in, 2 out]
            n138 = case shown="\"\"" w257 {
              tunnel: "TestMode/TestProgress" ("Name") -> [w270 _]
              tunnel: "TestMode/TestProgressText" ("Name") -> [w269 _]
              frame Default {
                n139 = call <vilib>:"NT Read Number.vi"("Name"=w270) -> ("Numeric"=w271:dbl)  [unwired: 9 in, 1 out]
                n140 = call <vilib>:"NT Read String.vi"("Name"=w269) -> ("String"=w272:string)  [unwired: 9 in, 1 out]
                n141 = Bundle("Numeric"=w271, "String"=w272) -> (→"Progress":cluster{"Numeric":dbl, "String":string})  [unwired: 1 in]
              }
              frame "" {
                n142 = property on="Progress" class="Clust (strict)"("Visible"=FALSE) -> ()  [unwired: 2 in, 2 out]
                n143 = local write "Test Name"(u16 0) -> ()
              }
            }
            n144 = property on="Test Tree" class="Tree (strict)"("Active Item Row Number"=w266, "ActiveColNum"=w266, "CellBG"=w263, "Active Item Row Number"=-1 ("Active Item:Row Number"), "CellBG"=u32 5789784 ("Color Box")) -> ()  [unwired: 2 in, 2 out]
          }
          frame "Variables" {
            w278 = string[] ["CameraPublisher", "Usage", "DB"]  # Items to initially close
            n145 = First Call?() -> (First Call?: T/F=w279:bool)
            n146 = control-ref of="Tree"() -> (w280:refnum<vi>)
            n147 = Select(t=w278, s=w279, f=string[] []) -> (s? t:f=w276:string[])
            n148 = call <vilib>:"NT Read and Format Entries as Tree.vi"("Tags to  Close"=w276, "Tree Refnum"=w280) -> ()  [unwired: 8 in, 2 out]
          }
          frame "Commands" {
            w289 = u32 5789784 ("Color Box")
            w290 = T26 {"Row"=-1, "Column"=-2} ("Active Cell:Active Cell")
            w292 = T26 {"Row"=-2, "Column"=-2} ("Active Cell:Active Cell")
            n149 = Index Array(array=w293, index=w287) -> (element=w291:u32)
            n150 = Index Array(array=w288, index=w287) -> (element=w286:T25)
            n151 = Unbundle(w286) -> ("Operation"=w285:enum16{"Update", "Clear"})  [unwired: 1 out]
            n152 = local read "Command Selection"() -> (w284:i32)
            n153 = property on="Command Selection" class="MCListbox (strict)"("ActiveCell"=w292, "CellBG"=w291, "ActiveCell"=w290, "CellBG"=w289) -> ()  [unwired: 2 in, 2 out]
            n154 = call <vilib>:"WPI_DashboardUpdate RPC Info.vi"("Operation"=w285) -> ("update"=w283:bool, "commands"=w282:string[][])  [unwired: 9 in]
            n155 = property on="Command Selection" class="MCListbox (strict)"("ItemNames"=w282) -> ()  [unwired: 2 in, 2 out]
            n156 = property on="Command Params" class="Tbl (strict)"("Active Cell"=w292, "Cell BG Color"=w291, "Active Cell"=w290, "Cell BG Color"=w289) -> ()  [unwired: 2 in, 2 out]
            n157 = call <vilib>:"WPI_DashboardUpdate Command Params.vi"("Update"=w283, "NewVal"=w284, "Commands"=w282, "Param Tbl"=w281) -> ()  [unwired: 7 in, 1 out]
          }
        }
        n158 = call <vilib>:"Connextion Info.vi"() -> ("Connected"=→"NT Connection":bool)  [unwired: 10 in, 1 out]
      }
      event "Test Tree": Value Change {
        # "Show appropriate\ncontrols"
        n159 = event-data() -> ("CtlRef"=w298:refnum<vi>, "NewVal"=w296:string)  [unwired: 1 in]
        n160 = call <vilib>:"WPI_UtilitiesGetTreeIOName.vi"("NewVal"=w296, "TreeControl in"=w298) -> ("I/O Name"=w299:string)  [unwired: 9 in]
        n161 = case shown="\"Camera\"" w299 {
          selector: w299 -> [_ w306 _ w328 w337 _]
          tunnel: w296 -> [_ _ w325 w327 _ w344]
          tunnel: cluster{string[]}[] [{["640x480", "320x240", "160x120"]}, {["Auto", "Fixed indoor", "Fixed outdoor 1", "Fixed outdoor 2", "Fixed fluorescent 1", "Fixed fluorescent 2", "Hold current"]}, {["Auto", "Flicker-free 50 Hz", "Flicker-free 60 Hz", "Hold current"]}, {["None", "Prioritize frame rate", "Prioritize image quality"]}, {["Monochrome", "Color"]}] -> [_ _ _ _ _ w343]
          frame Default {
            w301 = FALSE ("Visible")
            w300 = FALSE ("Visible")
            n162 = property on="Motor" class="Clust (strict)"("Visible"=w300) -> ()  [unwired: 2 in, 2 out]
            n163 = property on="Test Ring" class="Ring (strict)"("Visible"=w300) -> ()  [unwired: 2 in, 2 out]
            n164 = property on="Rev/Fwd" class="Clust (strict)"("Visible"=w301) -> ()  [unwired: 2 in, 2 out]
            n165 = property on="On/Off" class="Bool (strict)"("Visible"=w301) -> ()  [unwired: 2 in, 2 out]
            n166 = property on="Test Slider" class="Slide (strict)"("Visible"=w301) -> ()  [unwired: 2 in, 2 out]
          }
          frame "Analog Out", "Motor", "PWM" {
            w307 = FALSE ("Visible")
            n167 = case shown="\"Analog Out\"" w306 {
              tunnel: [1.0 ("Value") -1.0 ("Value") 0.0 ("Value")] -> w305
              tunnel: [255.0 ("Value") 1.0 ("Value") 5.0 ("Value")] -> w304
              tunnel: [128.0 ("Value") 0.0 ("Value") 0.0 ("Value")] -> w303
              tunnel: [64.0 ("Value") 0.5 ("Value") 1.0 ("Value")] -> w302
              frame "PWM" {
              }
              frame "Motor", Default {
              }
              frame "Analog Out" {
              }
            }
            n168 = property on="Motor" class="Clust (strict)"("Visible"=TRUE) -> ()  [unwired: 2 in, 2 out]
            n169 = property on="Value" class="Slide (strict)"("Value"=w303, "Scale.Minimum"=w305, "Scale.Maximum"=w304, "Scale.Increment"=w302) -> ()  [unwired: 2 in, 2 out]
            n170 = property on="On/Off" class="Bool (strict)"("Visible"=w307) -> ()  [unwired: 2 in, 2 out]
            n171 = property on="Test Slider" class="Slide (strict)"("Visible"=w307) -> ()  [unwired: 2 in, 2 out]
            n172 = property on="Test Ring" class="Ring (strict)"("Visible"=w307) -> ()  [unwired: 2 in, 2 out]
            n173 = property on="Rev/Fwd" class="Clust (strict)"("Visible"=w307) -> ()  [unwired: 2 in, 2 out]
          }
          frame "Servo" {
            w323 = FALSE ("Visible")
            n174 = call <vilib>:"NT Read Number.vi"("Name"=w325) -> ("Numeric"=w324:dbl)  [unwired: 9 in, 1 out]
            n175 = property on="Test Slider" class="Slide (strict)"("Visible"=TRUE, "Scale.Maximum"=170.0 ("Scale.Range:Maximum")) -> ()  [unwired: 2 in, 2 out]
            n176 = local write "Test Slider"(w324) -> ()
            n177 = property on="Motor" class="Clust (strict)"("Visible"=w323) -> ()  [unwired: 2 in, 2 out]
            n178 = property on="Rev/Fwd" class="Clust (strict)"("Visible"=w323) -> ()  [unwired: 2 in, 2 out]
            n179 = property on="On/Off" class="Bool (strict)"("Visible"=w323) -> ()  [unwired: 2 in, 2 out]
            n180 = property on="Test Ring" class="Ring (strict)"("Visible"=w323) -> ()  [unwired: 2 in, 2 out]
          }
          frame "Relay", "Solenoid" {
            w326 = FALSE ("Visible")
            n181 = property on="Motor" class="Clust (strict)"("Visible"=w326) -> ()  [unwired: 2 in, 2 out]
            n182 = property on="Test Slider" class="Slide (strict)"("Visible"=w326) -> ()  [unwired: 2 in, 2 out]
            n183 = Search and Replace String(input string=w327, search string="/Value  **", replace string="/Direction") -> (result string=w333:string)  [unwired: 5 in, 3 out]
            n184 = property on="Test Ring" class="Ring (strict)"("Visible"=w326) -> ()  [unwired: 2 in, 2 out]
            n185 = call <vilib>:"NT Read String.vi"("Name"=w333) -> ("String"=w331:string)  [unwired: 9 in, 1 out]
            n186 = Equal?(x="Both directions", y=w331) -> (x = y?=w329:bool)
            n187 = Not(x=w329) -> (.not. x?=w330:bool)
            n188 = property on="Rev/Fwd" class="Clust (strict)"("Visible"=w329) -> ()  [unwired: 2 in, 2 out]
            n189 = property on="On/Off" class="Bool (strict)"("Visible"=w330, "Caption.Text"=w328) -> ()  [unwired: 2 in, 2 out]
          }
          frame "Compressor", "Digital Out" {
            w336 = FALSE ("Visible")
            # "Get direction and finish"
            n190 = property on="Motor" class="Clust (strict)"("Visible"=w336) -> ()  [unwired: 2 in, 2 out]
            n191 = property on="Test Slider" class="Slide (strict)"("Visible"=w336) -> ()  [unwired: 2 in, 2 out]
            n192 = property on="Test Ring" class="Ring (strict)"("Visible"=w336) -> ()  [unwired: 2 in, 2 out]
            n193 = property on="On/Off" class="Bool (strict)"("Visible"=TRUE, "Caption.Text"=w337) -> ()  [unwired: 2 in, 2 out]
            n194 = property on="Rev/Fwd" class="Clust (strict)"("Visible"=FALSE) -> ()  [unwired: 2 in, 2 out]
          }
          frame "Camera" {
            n195 = call <vilib>:"Get Last Path Segment.vi"("String in"=w344) -> ("String out"=w345:string)  [unwired: 10 in]
            n196 = property on="On/Off" class="Bool (strict)"("Visible"=FALSE) -> ()  [unwired: 2 in, 2 out]
            n197 = property on="Motor" class="Clust (strict)"("Visible"=FALSE) -> ()  [unwired: 2 in, 2 out]
            n198 = property on="Rev/Fwd" class="Clust (strict)"("Visible"=FALSE) -> ()  [unwired: 2 in, 2 out]
            n199 = case shown="\"White Balance  **\"" w345 {
              tunnel: w344 -> [w351 w360 w369 w378 w387 _ w393]
              tunnel: w343 -> [w349 w357 w366 w375 w384 _ _]
              frame "Size  **" {
                n200 = Index Array(array=w349) -> (element=w348:cluster{string[]})  [unwired: 1 in]
                n201 = call <vilib>:"NT Read String.vi"("Name"=w351) -> ("String"=w350:string)  [unwired: 9 in, 1 out]
                n202 = Unbundle(w348) -> (w346:string[])
                n203 = Match First String(2:w346, 3:w350) -> (0:w347:i32)  [unwired: 1 out]
                n204 = property on="Test Ring" class="Ring (strict)"("Value"=w347, "Strings []"=w346) -> ()  [unwired: 2 in, 2 out]
                n205 = property on="Test Ring" class="Ring (strict)"("Visible"=TRUE) -> ()  [unwired: 2 in, 2 out]
                n206 = property on="Test Slider" class="Slide (strict)"("Visible"=FALSE) -> ()  [unwired: 2 in, 2 out]
              }
              frame "White Balance  **" {
                n207 = Index Array(array=w357, index=1) -> (element=w358:cluster{string[]})
                n208 = call <vilib>:"NT Read String.vi"("Name"=w360) -> ("String"=w359:string)  [unwired: 9 in, 1 out]
                n209 = Unbundle(w358) -> (w355:string[])
                n210 = Match First String(2:w355, 3:w359) -> (0:w354:i32)  [unwired: 1 out]
                n211 = property on="Test Ring" class="Ring (strict)"("Value"=w354, "Strings []"=w355) -> ()  [unwired: 2 in, 2 out]
                n212 = property on="Test Ring" class="Ring (strict)"("Visible"=TRUE) -> ()  [unwired: 2 in, 2 out]
                n213 = property on="Test Slider" class="Slide (strict)"("Visible"=FALSE) -> ()  [unwired: 2 in, 2 out]
              }
              frame "Exposure  **" {
                n214 = Index Array(array=w366, index=2) -> (element=w367:cluster{string[]})
                n215 = call <vilib>:"NT Read String.vi"("Name"=w369) -> ("String"=w368:string)  [unwired: 9 in, 1 out]
                n216 = Unbundle(w367) -> (w363:string[])
                n217 = Match First String(2:w363, 3:w368) -> (0:w364:i32)  [unwired: 1 out]
                n218 = property on="Test Ring" class="Ring (strict)"("Value"=w364, "Strings []"=w363) -> ()  [unwired: 2 in, 2 out]
                n219 = property on="Test Ring" class="Ring (strict)"("Visible"=TRUE) -> ()  [unwired: 2 in, 2 out]
                n220 = property on="Test Slider" class="Slide (strict)"("Visible"=FALSE) -> ()  [unwired: 2 in, 2 out]
              }
              frame "Exposure Priority  **" {
                n221 = Index Array(array=w375, index=3) -> (element=w376:cluster{string[]})
                n222 = call <vilib>:"NT Read String.vi"("Name"=w378) -> ("String"=w377:string)  [unwired: 9 in, 1 out]
                n223 = Unbundle(w376) -> (w372:string[])
                n224 = Match First String(2:w372, 3:w377) -> (0:w373:i32)  [unwired: 1 out]
                n225 = property on="Test Ring" class="Ring (strict)"("Value"=w373, "Strings []"=w372) -> ()  [unwired: 2 in, 2 out]
                n226 = property on="Test Ring" class="Ring (strict)"("Visible"=TRUE) -> ()  [unwired: 2 in, 2 out]
                n227 = property on="Test Slider" class="Slide (strict)"("Visible"=FALSE) -> ()  [unwired: 2 in, 2 out]
              }
              frame "Color Enable  **" {
                n228 = Index Array(array=w384, index=4) -> (element=w385:cluster{string[]})
                n229 = call <vilib>:"NT Read String.vi"("Name"=w387) -> ("String"=w386:string)  [unwired: 9 in, 1 out]
                n230 = Unbundle(w385) -> (w381:string[])
                n231 = Match First String(2:w381, 3:w386) -> (0:w382:i32)  [unwired: 1 out]
                n232 = property on="Test Ring" class="Ring (strict)"("Value"=w382, "Strings []"=w381) -> ()  [unwired: 2 in, 2 out]
                n233 = property on="Test Ring" class="Ring (strict)"("Visible"=TRUE) -> ()  [unwired: 2 in, 2 out]
                n234 = property on="Test Slider" class="Slide (strict)"("Visible"=FALSE) -> ()  [unwired: 2 in, 2 out]
              }
              frame Default {
                n235 = property on="Test Ring" class="Ring (strict)"("Visible"=FALSE) -> ()  [unwired: 2 in, 2 out]
                n236 = property on="Test Slider" class="Slide (strict)"("Visible"=FALSE) -> ()  [unwired: 2 in, 2 out]
              }
              frame "Brightness  **", "Color Level  **", "Compression  **", "FPS  **", "Sharpness  **" {
                n237 = call <vilib>:"NT Read Number.vi"("Name"=w393) -> ("Numeric"=w392:dbl)  [unwired: 9 in, 1 out]
                n238 = local write "Test Slider"(w392) -> ()
                n239 = property on="Test Slider" class="Slide (strict)"("Visible"=TRUE, "Scale.Maximum"=100.0 ("Scale.Range:Maximum")) -> ()  [unwired: 2 in, 2 out]
                n240 = property on="Test Ring" class="Ring (strict)"("Visible"=FALSE) -> ()  [unwired: 2 in, 2 out]
              }
            }
          }
        }
        n241 = property on="Progress" class="Clust (strict)"("Visible"=FALSE) -> ()  [unwired: 2 in, 2 out]
      }
      event "Test Name": Mouse Enter {
        # "Populate the ring with the list of tests"
        n242 = event-data() -> ()  [unwired: 1 in, 1 out]
        n243 = call <vilib>:"NT Read String Array.vi"("Name"="TestMode/TestList") -> ("String Array"=w401:string[])  [unwired: 9 in, 1 out]
        n244 = Build Array (concatenate)("Select the test to run...", w401) -> (w400:string[])
        n245 = property on="Test Name" class="Ring (strict)"("Strings []"=w400) -> ()  [unwired: 2 in, 2 out]
      }
      event "Test Name": Value Change {
        w403 = FALSE ("Visible")
        # "Tell the robot the test name to run"
        n246 = event-data() -> ("NewVal"=w407:u16)  [unwired: 1 in]
        n247 = property on="Test Name" class="Ring (strict)"() -> ("Strings []"=w408:string[])  [unwired: 2 in, 2 out]
        n248 = local write "Progress"(T6 {"Test Progress"=0, "Test Progress Text"=""} ("Progress")) -> ()
        n249 = Index Array(array=w408, index=w407) -> (element=w406:string)
        n250 = call <vilib>:"NT Write String.vi"("String"=w406, "Name"="TestMode/TestName") -> ()  [unwired: 9 in, 1 out]
        n251 = property on="Progress" class="Clust (strict)"("Visible"=TRUE) -> ()  [unwired: 2 in, 2 out]
        n252 = property on="Motor" class="Clust (strict)"("Visible"=w403) -> ()  [unwired: 2 in, 2 out]
        n253 = property on="Test Slider" class="Slide (strict)"("Visible"=w403) -> ()  [unwired: 2 in, 2 out]
        n254 = property on="On/Off" class="Bool (strict)"("Visible"=w403) -> ()  [unwired: 2 in, 2 out]
        n255 = property on="Rev/Fwd" class="Clust (strict)"("Visible"=w403) -> ()  [unwired: 2 in, 2 out]
        n256 = property on="Test Ring" class="Ring (strict)"("Visible"=w403) -> ()  [unwired: 2 in, 2 out]
      }
      event "Select Auto": Mouse Enter {
        # "Populate the combo box with the list of autonomous options"
        n257 = event-data() -> ()  [unwired: 1 in, 1 out]
        n258 = call <vilib>:"NT Read String Array.vi"("Name"="Auto List") -> ("String Array"=w410:string[])  [unwired: 9 in, 1 out]
        n259 = property on="Select Auto" class="CmbBox"("Strings[]"=w410) -> ()  [unwired: 2 in, 2 out]
      }
      event "Select Auto": Value Change {
        # "User modified the Auto Selection. Write to NT variable so robot knows."
        n260 = event-data() -> ("NewVal"=w413:string)  [unwired: 1 in]
        n261 = call <vilib>:"NT Write String.vi"("String"=w413, "Name"="Auto Selector") -> ()  [unwired: 9 in, 1 out]
      }
      event "Command Selection": Value Change {
        # "Get the params and show in table"
        n262 = event-data() -> ("NewVal"=w419:i32)  [unwired: 1 in]
        n263 = property on="Command Selection" class="MCListbox (strict)"() -> ("ItemNames"=w417:string[][])  [unwired: 2 in, 2 out]
        n264 = call <vilib>:"WPI_DashboardUpdate Command Params.vi"("NewVal"=w419, "Commands"=w417, "Param Tbl"=w418) -> ()  [unwired: 8 in, 1 out]
      }
      event "Execute Command": Value Change {
        # "Started one, Unique ID holds\nresponse"
        n265 = event-data() -> ()  [unwired: 1 in, 1 out]
        n266 = property on="Command Selection" class="MCListbox (strict)"() -> ("ItemNames"=w430:string[][])  [unwired: 2 in, 2 out]
        n267 = Index Array(array=w430, index (row)="Command Selection", index (col)=0) -> (element=w428:string)
        n268 = call <vilib>:"Invoke Commands.vi"("Command Params"="Command Params", "Function Name"=w428) -> ("Params"=w424:u8, "Started"=w423:bool)  [unwired: 7 in, 1 out]
        n269 = Array Subset(array="Command Params", length (row)=w424) -> (w425:string[][])  [unwired: 3 in]
        n270 = Select(t="Executing" ("Cmd Status"), s=w423, f="" ("Cmd Status")) -> (s? t:f=→"Cmd Status":string)
      }
      event "Command Selection": Double Click {
        n271 = event-data() -> ("Row"=w438:i32)  [unwired: 1 in]
        n272 = property on="Command Selection" class="MCListbox (strict)"() -> ("ItemNames"=w441:string[][])  [unwired: 2 in, 2 out]
        n273 = local read "Command Params"() -> (w437:string[][])
        n274 = Index Array(array=w441, index (row)=w438, index (col)=0) -> (element=w439:string)
        n275 = call <vilib>:"Invoke Commands.vi"("Command Params"=w437, "Function Name"=w439) -> ("Params"=w436:u8, "Started"=w431:bool)  [unwired: 7 in, 1 out]
        n276 = Array Subset(array=w437, length (row)=w436) -> (w435:string[][])  [unwired: 3 in]
        n277 = Select(t="Executing" ("Cmd Status"), s=w431, f="" ("Cmd Status")) -> (s? t:f=w432:string)
        n278 = local write "Cmd Status"(w432) -> ()
      }
      event "CheckList": Double Click {
        # "Shift clears all"
        # "Update symbols on the listbox"
        n279 = event-data() -> ("PlatMods.Shift"=w443:bool, "Row"=w445:i32)  [unwired: 1 in]
        n280 = case shown="True" w443 {
          tunnel: w445 -> [w449 _]
          tunnel: 1 -> [w448 _]
          frame False {
            n281 = property on="CheckList" class="LstBox (strict)"() -> ("Item Symbols"=w447:i32[])  [unwired: 2 in, 2 out]
            n282 = Replace Array Subset(array=w447, new element=w448, index=w449) -> (w446:i32[])
            n283 = property on="CheckList" class="LstBox (strict)"("Item Symbols"=w446) -> ()  [unwired: 2 in, 2 out]
          }
          frame True {
            w450 = 0 ("Top Row")
            n284 = property on="CheckList" class="LstBox (strict)"() -> ("Number of Rows"=w452:u32)  [unwired: 2 in, 2 out]
            n285 = Initialize Array(0, w452) -> (w451:i32[])
            n286 = property on="CheckList" class="LstBox (strict)"("Top Row"=w450, "Value"=w450, "Item Symbols"=w451) -> ()  [unwired: 2 in, 2 out]
          }
        }
      }
      event "CheckList": Key Down {
        # "Update symbols on the listbox\nLeft and right keys check and uncheck"
        n287 = event-data() -> ("VKey"=w456:T23)  [unwired: 1 in]
        n288 = case shown="\"Left\", \"Right\"" w456 {
          selector: w456 -> [w461 _]
          tunnel: eventvkey."Left" ("VKey") -> [w459 _]
          frame "Left", "Right" {
            n289 = Equal?(x=w459, y=w461) -> (x = y?=w460:bool)
            n290 = Select(t=0, s=w460, f=1) -> (s? t:f=w462:i32)
            n291 = property on="CheckList" class="LstBox (strict)"() -> ("Item Symbols"=w465:i32[])  [unwired: 2 in, 2 out]
            n292 = Replace Array Subset(array=w465, new element=w462, index="CheckList") -> (w464:i32[])
            n293 = property on="CheckList" class="LstBox (strict)"("Item Symbols"=w464) -> ()  [unwired: 2 in, 2 out]
          }
          frame Default {
          }
        }
      }
      event "Motor.Enable": Value Change {
        # "When the test mode otor enable helper is set, update that\ntree row item's value"
        n294 = event-data() -> ("NewVal"=w471:bool)  [unwired: 1 in]
        n295 = Unbundle("Motor") -> ("Value"=w470:dbl)  [unwired: 1 out]
        n296 = Select(t=w470, s=w471, f=0.0) -> (s? t:f=w468:dbl)
        n297 = call <vilib>:"NT Write Number.vi"("Numeric"=w468, "Name"=w467) -> ()  [unwired: 9 in, 1 out]
      }
      event "Test Slider": Value Change {
        # "When the test mode slider helper is set, update that\ntree row item's value"
        n298 = event-data() -> ("NewVal"=w474:dbl)  [unwired: 1 in]
        n299 = call <vilib>:"NT Write Number.vi"("Numeric"=w474, "Name"=w475) -> ()  [unwired: 9 in, 1 out]
      }
      event "On/Off": Value Change {
        # "When the test mode on/off helper value is set, update that\ntree row item's value"
        n300 = event-data() -> ("NewVal"=w479:bool)  [unwired: 1 in]
        n301 = Boolean To (0,1)(Boolean=w479) -> (0, 1=w478:i16)
        n302 = call <vilib>:"NT Write Number.vi"("Numeric"=w478, "Name"=w477) -> ()  [unwired: 9 in, 1 out]
      }
      event "Rev/Fwd": Value Change {
        # "When the test mode helper value for relays is set, update that\ntree row item's value"
        n303 = event-data() -> ("NewVal.Forward"=w487:bool, "NewVal.Reverse"=w486:bool)  [unwired: 1 in]
        n304 = Boolean To (0,1)(Boolean=w487) -> (0, 1=w483:i16)
        n305 = Boolean To (0,1)(Boolean=w486) -> (0, 1=w485:i16)
        n306 = Negate(x=w485) -> (-x=w484:i16)
        n307 = Add(x=w483, y=w484) -> (x+y=w482:i16)
        n308 = call <vilib>:"NT Write Number.vi"("Numeric"=w482, "Name"=w481) -> ()  [unwired: 9 in, 1 out]
      }
      event "Test Ring": Value Change {
        # "When a test mode helper value is selected from the ring,\nset the tree item's variable to the string value"
        n309 = event-data() -> ("NewVal"=w491:u16)  [unwired: 1 in]
        n310 = property on="Test Ring" class="Ring (strict)"() -> ("Strings []"=w492:string[])  [unwired: 2 in, 2 out]
        n311 = Index Array(array=w492, index=w491) -> (element=w490:string)
        n312 = call <vilib>:"NT Write String.vi"("String"=w490, "Name"=w489) -> ()  [unwired: 9 in, 1 out]
      }
      event "Rec Mode": Value Change {
        # "Update globals for recording mode and path to read log from.\nClear when logging and let NetworkTables set path for vision to\nuse."
        n313 = event-data() -> ("NewVal"=w503:enum32{"Stop", "Record", "Playback"})  [unwired: 1 in]
        n314 = global write "WPI_DashboardLogging Global.vi" "Logging Filename"(path "") -> ()
        n315 = global write "WPI_DashboardLogging Global.vi" "Recording"(w503) -> ()
        n316 = case shown="\"Playback\"" w503 {
          tunnel: w502 -> [_ w505 w514]
          tunnel: [_ _ w513] -> w500
          tunnel: [_ _ w512] -> _
          tunnel: w498 -> [_ _ w510]
          tunnel: cluster{i32, i32} {-250, 170} -> [_ _ w509]
          tunnel: [_ _ T24 {"Image Size"=TRUE, "Image Type"=TRUE, "Pixel Value"=TRUE, "ROI Information"=TRUE, "Zoom Factor"=FALSE} ("Image Information Shown:All Elements")] -> w493
          tunnel: [_ _ TRUE ("Zoom Factor")] -> w494
          tunnel: w496 -> [_ _ w506]
          frame Default {
          }
          frame "Stop", "Record" {
            # "Place Window too"
            n317 = invoke class="VI" method="FP.Close"(reference=w505) -> (reference out=w504:refnum<vi>)  [unwired: 2 in, 2 out]
            n318 = invoke class="VI" method="Abort VI"(reference=w504) -> ()  [unwired: 2 in, 3 out]
          }
          frame "Playback" {
            n319 = call "Open Playback Panel.vi"("Offset"=w509, "DB VI Ref"=w510, "Playback in"=w514) -> ("Playback out"=w511:refnum<vi>)  [unwired: 8 in]
            n320 = register-events(w511, w506) -> (reference out=w513:refnum<event-registration>, error out=w512:errorcluster)  [unwired: 2 in]
          }
        }
        n321 = property on="Camera Image Right" class="ImageControl"("Image Information Shown"=w493, "Image Information Visible"=w494) -> ()  [unwired: 2 in, 2 out]
        n322 = property on="Camera Image" class="ImageControl"("Image Information Shown"=w493, "Image Information Visible"=w494) -> ()  [unwired: 2 in, 2 out]
        n323 = call <vilib>:"WPI_DashboardNT Log FieldName Cache.vi"("Operation"=enum16{"Lookup/Add", "Index", "Clear"}."Clear") -> ()  [unwired: 8 in, 3 out]
      }
      event Panel Close {
        w516 = enum32{"Stop", "Record", "Playback"}."Stop" ("Rec Mode")
        # "Playback window has been closed, abort"
        n324 = event-data() -> ()  [unwired: 1 in, 4 out]
        n325 = local write "Rec Mode"(w516) -> ()
        n326 = global write "WPI_DashboardLogging Global.vi" "Recording"(w516) -> ()
      }
      event Panel Close {
        # "Abort playback window and ourself"
        n327 = event-data() -> ()  [unwired: 1 in, 4 out]
        n328 = invoke class="VI" method="FP.Close"(reference=w520) -> (reference out=w519:refnum<vi>)  [unwired: 2 in, 2 out]
        n329 = invoke class="VI" method="Abort VI"(reference=w519) -> (error out=w518:errorcluster)  [unwired: 2 in, 2 out]
        n330 = invoke class="VI" method="Abort VI"(error in=w518) -> ()  [unwired: 2 in, 3 out]
      }
      event User Event {
        n331 = event-data() -> ("IDs"=w527:cluster{"RPC field ID":u16, "Unique ID":u16}, "String"=w526:string)  [unwired: 1 in]
        n332 = Bundle("IDs"=w527, "String"=w526) -> (w525:T10)  [unwired: 1 in]
        n333 = call <vilib>:"Retrieve RPC Response.vi"("RPC Response"=w525) -> ("Output"=w523:string[][])  [unwired: 10 in]
        n334 = Build Array (concatenate)(w521, w523) -> (w522:string[][])
        n335 = local write "Command Params"(w522) -> ()
        n336 = local write "Cmd Status"("" ("Cmd Status")) -> ()
      }
      event "Tree": Double Click {
        n337 = event-data() -> ("PlatMods"=w533:T27, "Tag"=w530:string)  [unwired: 1 in]
        n338 = Unbundle(w533) -> ("Shift"=w532:bool)  [unwired: 4 out]
        n339 = String Subset(string=w530, length (rest)=1 ("length (rest)")) -> (substring=w529:string)  [unwired: 1 in]
        n340 = Not(x=w532) -> (.not. x?=w531:bool)
        n341 = case shown="\"/\"" w529 {
          tunnel: w530 -> [_ w536]
          tunnel: w531 -> [_ w535]
          frame Default {
          }
          frame "/" {
            n342 = call <vilib>:"NT Update Persistence.vi"("Persistence"=w535, "Name"=w536) -> ()  [unwired: 9 in, 1 out]
          }
        }
      }
    }
  }
  n343 = while {
    tunnel: w65 -> [w538]
    i -> [w541]
    stop <- FALSE stop-if-true
    n344 = Wait (ms)(milliseconds to wait=u32 100) -> ()  [unwired: 1 out]
    n345 = case shown="\"Playback\"" "Rec Mode" {
      tunnel: w541 -> [_ _ w556]
      tunnel: [u32 2829099 ("Base Color") u32 11141120 ("Target Color") w545] -> w537
      frame "Stop", Default {
        # "Reset the color, extra updates don't cost much"
      }
      frame "Record" {
      }
      frame "Playback" {
        # "Playback"
        n346 = Quotient & Remainder(x=w556, y=u32 50 ("milliseconds to wait")) -> (x-y*floor(x/y)=w552:u32)  [unwired: 1 out]
        n347 = Divide(x=w552, y=u32 50 ("milliseconds to wait")) -> (x/y=w549:dbl)
        n348 = Multiply(x=6.283185307179586, y=w549) -> (x*y=w554:dbl)
        n349 = Sine(x=w554) -> (sin(x)=w553:dbl)
        n350 = Absolute Value(x=w553) -> (abs(x)=w546:dbl)
        n351 = call "Interpolate RGB Color.vi"("Proportion"=w546, "Target Color"=u32 30976, "Base Color"=u32 2829099) -> ("Result Color"=w545:u32)  [unwired: 8 in]
      }
    }
    n352 = property class="Pane"(reference=w538, "PaneColor"=w537) -> ()  [unwired: 1 in, 2 out]
  }
  n353 = local write "Dashboard Tab"(T8."Drive" ("Dashboard Tab")) -> ()
  n354 = property on="On/Off" class="Bool (strict)"("Visible"=w36) -> ()  [unwired: 2 in, 2 out]
  n355 = property on="Motor" class="Clust (strict)"("Visible"=w36) -> ()  [unwired: 2 in, 2 out]
  n356 = property on="Progress" class="Clust (strict)"("Visible"=w36) -> ()  [unwired: 2 in, 2 out]
  n357 = property on="Test Ring" class="Ring (strict)"("Visible"=w36) -> ()  [unwired: 2 in, 2 out]
  n358 = property on="Rev/Fwd" class="Clust (strict)"("Visible"=w36) -> ()  [unwired: 2 in, 2 out]
  n359 = while {
    tunnel: u16 1741 ("timeout ms (25000)") -> [w558]
    stop <- FALSE stop-if-true
    n360 = TCP Create Listener(10:w558) -> (0:w557:errorcluster, 3:w559:refnum<k5>)  [unwired: 4 in, 1 out]
    n361 = case shown="No Error" w557 {
      selector: w557 -> [w561 _]
      tunnel: w559 -> [w562 _]
      frame No Error {
        n362 = while {
          tunnel: w562 -> [w565]
          tunnel: w561 -> [w564]
          stop <- FALSE stop-if-true
          n363 = TCP Wait On Listener(8:w564, 11:w565) -> (0:w566:errorcluster, 4:w567:refnum<k5>)  [unwired: 2 in, 3 out]
          n364 = local write "TCP"(w567) -> ()
          n365 = case shown="No Error" w566 {
            frame No Error {
            }
            frame Error {
              n366 = Wait (ms)(milliseconds to wait=u32 1000) -> ()  [unwired: 1 out]
            }
          }
        }
      }
      frame Error {
        n367 = Wait (ms)(milliseconds to wait=u32 1000) -> ()  [unwired: 1 out]
      }
    }
  }
  n368 = local write "Command Selection"(u16 0 ("milliseconds to wait")) -> ()
  n369 = local write "Command Params"(string[][] [] ("Command Params")) -> ()
  n370 = global write "WPI_DashboardLogging Global.vi" "Recording"(w59) -> ()
  n371 = local write "Rec Mode"(w59) -> ()
  n372 = call <vilib>:"NT Write String.vi"("String"="Select Auto", "Name"="Auto Selector") -> ()  [unwired: 9 in, 1 out]
